vi "experiment description to file name Gershow.vi"(6 "use short dir":bool, 7 "Training/Habituation Pre Exposure":T2, 8 "error in":errorcluster, 9 "Stimulus Array":T1(array[cluster]), 10 "Genotype":T3={"GAL4 Line / Line A / Genotype"="CS", "UAS-Effector Line / Line B"=""}, 11 "Project":string) -> (0 "error out":errorcluster, 1 "data directory with time":path, 2 "filename":string, 3 "data directory":path)   [LabVIEW 2021]
panel:
  # "X"
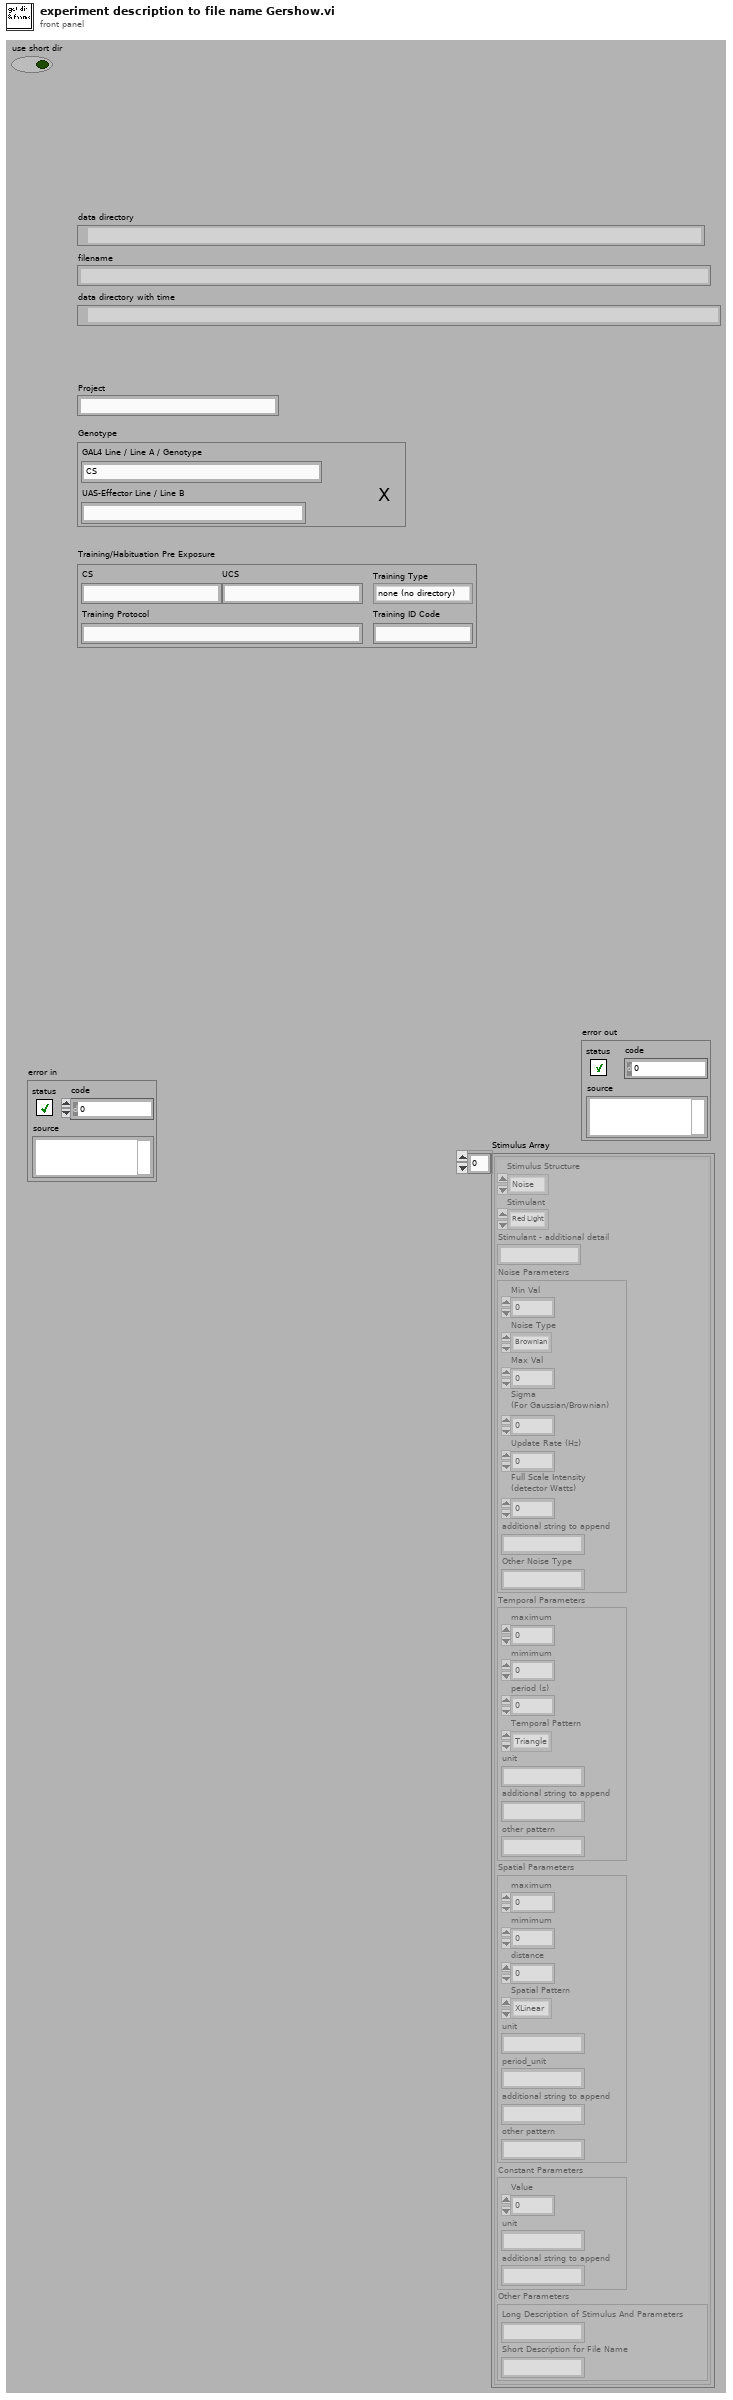
[diagram p1: front panel]
types:
  T1 = cluster{"Stimulus Structure":enum16{"Noise", "Temporal", "Spatial", "Constant", "Other"}, "Stimulant":enum16{"Red Light", "Blue Light", "Green Light", "Odor", "Temperature", "Taste", "Other"}, "Stimulant - additional detail":string, "Noise Parameters":cluster{"Min Val":dbl, "Noise Type":enum16{"Brownian", "Gaussian", "M-Sequence", "Integral of M-Sequence", "Bernoulli", "Uniform", "Other"}, "Max Val":dbl, "Sigma \n(For Gaussian/Brownian)":dbl, "Update Rate (Hz)":dbl, "Full Scale Intensity \n(detector Watts)":dbl, "additional string to append":string, "Other Noise Type":string}, "Temporal Parameters":cluster{"maximum":dbl, "mimimum":dbl, "period (s)":dbl, "Temporal Pattern":enum16{"Triangle", "Sine", "Square", "Other"}, "unit":string, "additional string to append":string, "other pattern":string}, "Spatial Parameters":cluster{"maximum":dbl, "mimimum":dbl, "distance":dbl, "Spatial Pattern":enum16{"XLinear", "YLinear", "Droplet", "Radial", "Other"}, "unit":string, "period_unit":string, "additional string to append":string, "other pattern":string}, "Constant Parameters":cluster{"Value":dbl, "unit":string, "additional string to append":string}, "Other Parameters":cluster{"Long Description of Stimulus And Parameters":string, "Short Description for File Name":string}}[]
  T2 = cluster{"CS":string, "UCS":string, "Training Protocol":string, "Training ID Code":string, "Training Type":enum16{"none (no directory)", "habituated", "mock habituated", "untrained", "trained"}}
  T3 = cluster{"GAL4 Line / Line A / Genotype":string, "UAS-Effector Line / Line B":string}
  T4 = enum16{"none (no directory)", "habituated", "mock habituated", "untrained", "trained"}
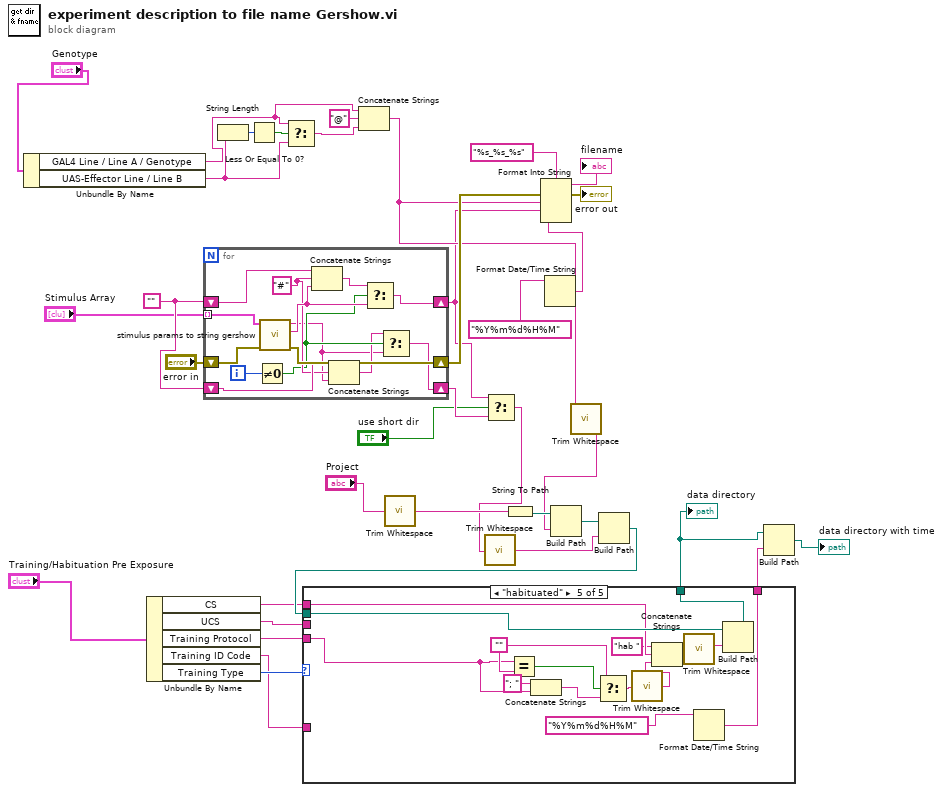
[diagram p0: block diagram]
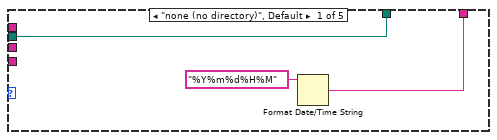
[diagram p2: hidden frame]
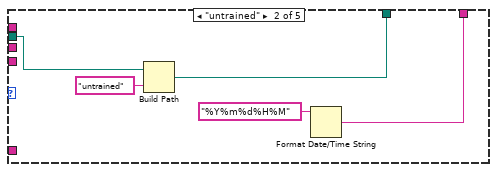
[diagram p3: hidden frame]
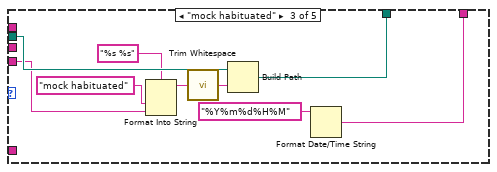
[diagram p4: hidden frame]
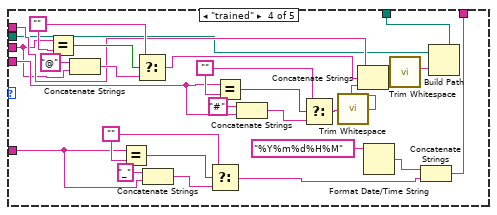
[diagram p5: hidden frame]
diagram:
  w24 = "" ("stimulus string description")
  n1 = Unbundle By Name("Genotype") -> ("GAL4 Line / Line A / Genotype"=w7:string, "UAS-Effector Line / Line B"=w14:string)
  n2 = Unbundle By Name("Training/Habituation Pre Exposure") -> ("CS"=w18:string, "UCS"=w6:string, "Training Protocol"=w17:string, "Training ID Code"=w5:string, "Training Type"=w23:T4)
  n3 = for {
    shift-right: [w50] -> w4
    shift-left: w24 -> [w49]
    shift-right: [w47] -> w35
    shift-left: "error in" -> [w46]
    shift-right: [w39] -> w3
    shift-left: w24 -> [w44]
    tunnel: "Stimulus Array" -> [w38] mode=indexing
    i -> [w51]
    w43 = "#"
    n4 = Not Equal To 0?(x=w51) -> (x != 0?=w42:bool)
    n5 = call "stimulus params to string gershow.vi"("error in"=w46, "Stimulus Cluster In"=w38) -> ("error out"=w47:errorcluster, "Short String"=w45:string, "Long String"=w40:string)  [unwired: 5 in, 2 out]
    n6 = Concatenate Strings(w49, w43, w45) -> (w48:string)
    n7 = Concatenate Strings(w44, w43, w40) -> (w41:string)
    n8 = Select(t=w48, s=w42, f=w45) -> (s? t:f=w50:string)
    n9 = Select(t=w41, s=w42, f=w40) -> (s? t:f=w39:string)
  }
  n10 = String Length(string=w14) -> (length=w27:i32)
  n11 = Less Or Equal To 0?(x=w27) -> (x <= 0?=w26:bool)
  n12 = Select(t=w7, s=w26, f=w14) -> (s? t:f=w16:string)
  n13 = Concatenate Strings(w7, "@" ("string"), w16) -> (w15:string)
  n14 = call <vilib>:"Trim Whitespace.vi"("string"="Project") -> ("trimmed string"=w13:string)  [unwired: 1 in]
  n15 = Select(t=w4, s="use short dir", f=w3) -> (s? t:f=w1:string)
  n16 = call <vilib>:"Trim Whitespace.vi"("string"=w1) -> ("trimmed string"=w12:string)  [unwired: 1 in]
  n17 = String To Path(string=w13) -> (path=w31:path)
  n18 = Format Date/Time String(time format string (%c)="%Y%m%d%H%M") -> (date/time string=w28:string)  [unwired: 2 in]
  n19 = Format Into String(format string="%s_%s_%s", error in=w35, w15, w4, w28) -> (resulting string=→"filename":string, error out=→"error out":errorcluster)  [unwired: 1 in]
  n20 = call <vilib>:"Trim Whitespace.vi"("string"=w15) -> ("trimmed string"=w11:string)  [unwired: 1 in]
  n21 = Build Path(base path=w31, name or relative path=w11) -> (appended path=w30:path)
  n22 = Build Path(base path=w30, name or relative path=w12) -> (appended path=w22:path)
  n23 = case shown="\"habituated\"" w23 {
    tunnel: w22 -> [w54 w59 w68 w78 w103]
    tunnel: [w54 w57 w67 w77 w102] -> w21
    tunnel: [w52 w55 w65 w73 w96] -> w20
    tunnel: w18 -> [_ _ _ w80 w99]
    tunnel: w17 -> [_ _ w61 w83 w106]
    tunnel: w6 -> [_ _ _ w70 _]
    tunnel: w5 -> [_ _ _ w69 _]
    frame "none (no directory)", Default {
      n24 = Format Date/Time String(time format string (%c)="%Y%m%d%H%M") -> (date/time string=w52:string)  [unwired: 2 in]
    }
    frame "untrained" {
      n25 = Build Path(base path=w59, name or relative path="untrained") -> (appended path=w57:path)
      n26 = Format Date/Time String(time format string (%c)="%Y%m%d%H%M") -> (date/time string=w55:string)  [unwired: 2 in]
    }
    frame "mock habituated" {
      n27 = Format Into String(format string="%s %s", "mock habituated" ("name or relative path"), w61) -> (resulting string=w64:string)  [unwired: 2 in, 1 out]
      n28 = call <vilib>:"Trim Whitespace.vi"("string"=w64) -> ("trimmed string"=w60:string)  [unwired: 1 in]
      n29 = Build Path(base path=w68, name or relative path=w60) -> (appended path=w67:path)
      n30 = Format Date/Time String(time format string (%c)="%Y%m%d%H%M") -> (date/time string=w65:string)  [unwired: 2 in]
    }
    frame "trained" {
      w85 = ""
      w89 = ""
      w93 = ""
      n31 = Equal?(x=w70, y=w93) -> (x = y?=w94:bool)
      n32 = Concatenate Strings("@" ("string"), w70) -> (w92:string)
      n33 = Equal?(x=w69, y=w89) -> (x = y?=w90:bool)
      n34 = Select(t=w93, s=w94, f=w92) -> (s? t:f=w81:string)
      n35 = Concatenate Strings("_" ("string"), w69) -> (w88:string)
      n36 = Select(t=w89, s=w90, f=w88) -> (s? t:f=w74:string)
      n37 = Equal?(x=w83, y=w85) -> (x = y?=w86:bool)
      n38 = Concatenate Strings("#" ("string"), w83) -> (w84:string)
      n39 = Select(t=w85, s=w86, f=w84) -> (s? t:f=w82:string)
      n40 = call <vilib>:"Trim Whitespace.vi"("string"=w82) -> ("trimmed string"=w72:string)  [unwired: 1 in]
      n41 = Concatenate Strings(w80, w81, w72) -> (w79:string)
      n42 = Format Date/Time String(time format string (%c)="%Y%m%d%H%M") -> (date/time string=w75:string)  [unwired: 2 in]
      n43 = call <vilib>:"Trim Whitespace.vi"("string"=w79) -> ("trimmed string"=w71:string)  [unwired: 1 in]
      n44 = Concatenate Strings(w75, w74) -> (w73:string)
      n45 = Build Path(base path=w78, name or relative path=w71) -> (appended path=w77:path)
    }
    frame "habituated" {
      w108 = ""
      n46 = Equal?(x=w106, y=w108) -> (x = y?=w109:bool)
      n47 = Concatenate Strings("; " ("string"), w106) -> (w107:string)
      n48 = Select(t=w108, s=w109, f=w107) -> (s? t:f=w105:string)
      n49 = call <vilib>:"Trim Whitespace.vi"("string"=w105) -> ("trimmed string"=w101:string)  [unwired: 1 in]
      n50 = Concatenate Strings("hab " ("string"), w99, w101) -> (w104:string)
      n51 = call <vilib>:"Trim Whitespace.vi"("string"=w104) -> ("trimmed string"=w100:string)  [unwired: 1 in]
      n52 = Format Date/Time String(time format string (%c)="%Y%m%d%H%M") -> (date/time string=w96:string)  [unwired: 2 in]
      n53 = Build Path(base path=w103, name or relative path=w100) -> (appended path=w102:path)
    }
  }
  "data directory" <- w21
  n54 = Build Path(base path=w21, name or relative path=w20) -> (appended path=→"data directory with time":path)
